vi "mj_localized.vi"(9 "TermSpecs":T1[](array[typedef]), 11 "Node type":T4(ring)) -> (2 "improperly localized?":bool)   [LabVIEW 2020]
uses:
  <vilib>/Platform/storage/lvStorage.llb/TerminalDef.ctl
  <vilib>/Platform/storage/lvStorage.llb/_TerminalStyle.ctl
  <vilib>/Utility/XNodeSupport.llb/XRect32.ctl
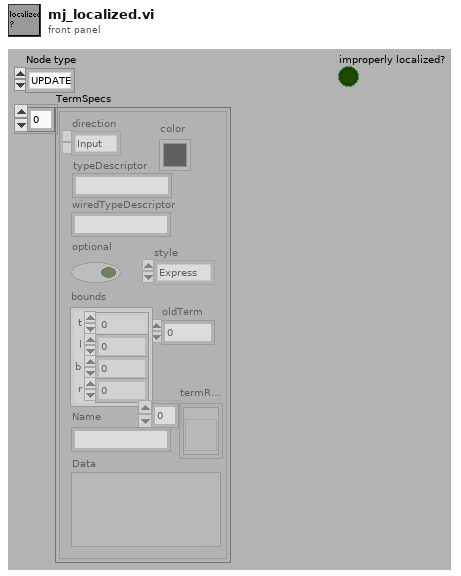
[diagram p1: front panel]
types:
  T1 = typedef "TerminalDef.ctl" = cluster{"direction":enum16{"Input", "Output"}, "typeDescriptor":string, "color":u32, "oldTerm":i32, "style":T2, "optional":bool, "bounds":T3, "termRefs":refnum<vi>[], "Name":string, "Data":variant, "wiredTypeDescriptor":string}
  T2 = typedef "_TerminalStyle.ctl" = enum16{"Express", "Collapsed", "Internal"}
  T3 = typedef "XRect32.ctl" = cluster{"t":i32, "l":i32, "b":i32, "r":i32}
  T4 = enum16{"UPDATE", "READ", "QUERY", "CREATE CHILD", "CREATE", "CONNECT", "DISCONNECT"}
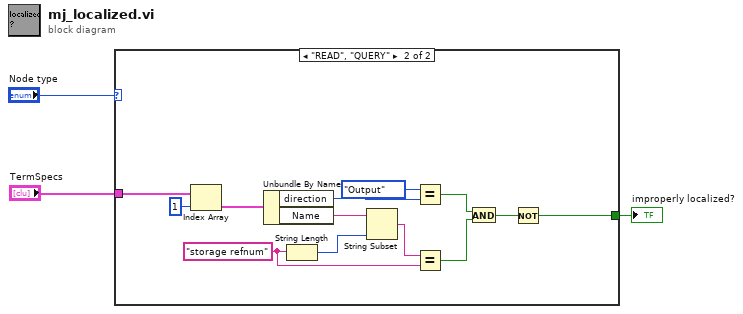
[diagram p0: block diagram]
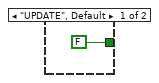
[diagram p2: hidden frame]
diagram:
  n1 = case shown="\"READ\", \"QUERY\"" "Node type" {
    tunnel: "TermSpecs" -> [_ w17]
    tunnel: [FALSE w5] -> w1
    frame "UPDATE", Default {
    }
    frame "READ", "QUERY" {
      w11 = "storage refnum" ("Name")
      n2 = Index Array(array=w17, index=1) -> (element=w15:T1)
      n3 = Unbundle By Name(w15) -> ("direction"=w10:enum16{"Input", "Output"}, "Name"=w14:string)
      n4 = String Length(string=w11) -> (length=w13:i32)
      n5 = String Subset(string=w14, length (rest)=w13) -> (substring=w12:string)  [unwired: 1 in]
      n6 = Equal?(x=enum16{"Input", "Output"}."Output", y=w10) -> (x = y?=w8:bool)
      n7 = Equal?(x=w12, y=w11) -> (x = y?=w7:bool)
      n8 = And(x=w8, y=w7) -> (x .and. y?=w6:bool)
      n9 = Not(x=w6) -> (.not. x?=w5:bool)
    }
  }
  "improperly localized?" <- w1
